vi "Close.vi"(8 "error in (no error)":errorcluster, 11 "PI650 VoltageAmp in":refnum<class "PI650 VoltageAmp.lvclass">) -> (0 "error out":errorcluster, 3 "PI650 VoltageAmp out":refnum<class "PI650 VoltageAmp.lvclass">)   [LabVIEW 2020, in "Pickering.lvlib" / "PI650 VoltageAmp.lvclass"]
uses:
  PI650 VoltageAmp.lvclass
  PI650 VoltageAmp.lvclass/PI650 VoltageAmp.ctl
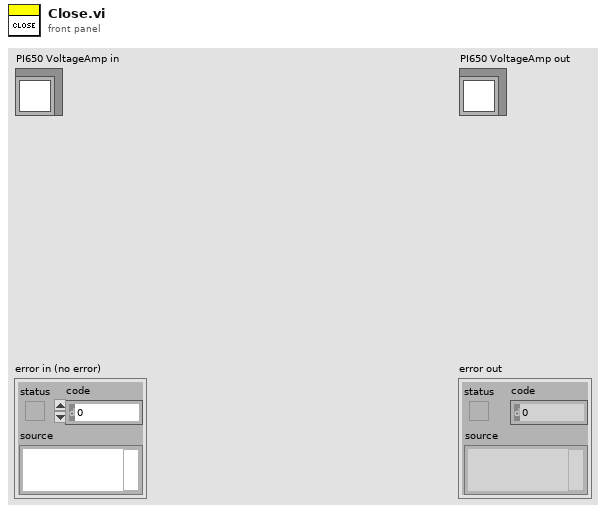
[diagram p1: front panel]
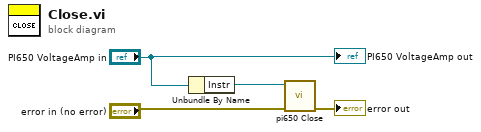
[diagram p0: block diagram]
diagram:
  n1 = Unbundle By Name("PI650 VoltageAmp in") -> ("Instr"=w2:refnum<visa-resource-name>)
  n2 = call <instrlib>:"pi650 Close.vi"("error in (no error)"="error in (no error)", "instrument handle"=w2) -> ("error out"=→"error out":errorcluster)  [unwired: 9 in]
  "PI650 VoltageAmp out" <- "PI650 VoltageAmp in"
